vi "start_sweep.vi"(8 "error in (no error)":errorcluster, 11 "DL090130ExperimentController in":refnum<class "ExperimentControllerDL090130Interval.lvclass">) -> (0 "error out":errorcluster, 3 "DL090130ExperimentController out":refnum<class "ExperimentControllerDL090130Interval.lvclass">)   [LabVIEW 2010, in "ExperimentControllerDL090130Interval.lvclass"]
uses:
  ExperimentControllerDL090130Interval.lvclass
  ExperimentControllerDL090130Interval.lvclass/ExperimentControllerDL090130Interval.ctl
  common/classes/ErrorController/ErrorController/class_data.vi
  ImagingMode/GenericImagingMode/GenericImagingMode/GenericImagingMode.lvclass
  common/classes/ErrorController/ErrorController/ErrorController.lvclass
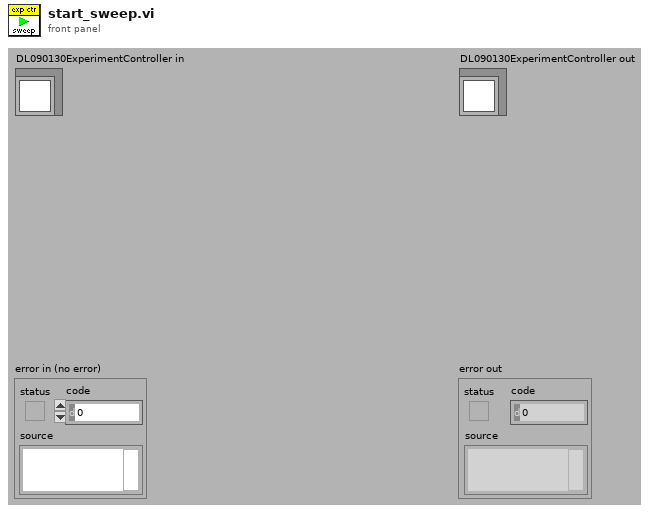
[diagram p1: front panel]
types:
  T1 = typedef "GenericToplevelComponent.lvclass/common_trigger_enum.ctl" = enum16{"NULL", "initialise", "terminate", "fetch command", "fetch data", "attach observer", "register as observer", "detach observer", "acknowledge", "start", "stop", "sweep started", "sweep finished", "experiment started", "experiment stopped"}
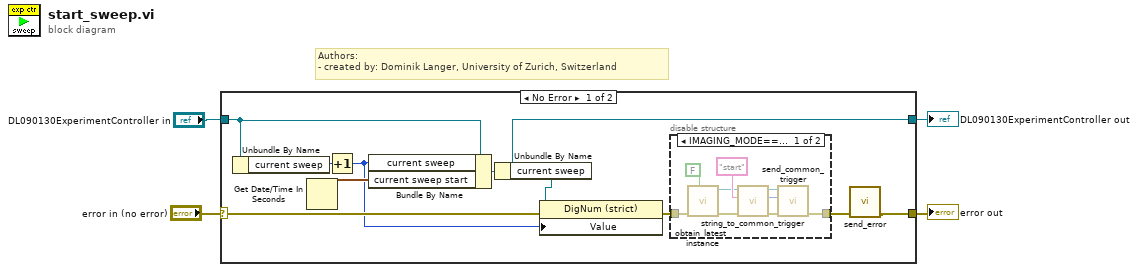
[diagram p0: block diagram]
diagram:
  # "Authors: \n- created by: Dominik Langer, University of Zurich, Switzerland"
  n1 = case shown="No Error" "error in (no error)" {
    selector: "error in (no error)" -> [w10 w26]
    tunnel: [w6 w26] -> w3
    tunnel: [w8 w25] -> w1
    tunnel: "DL090130ExperimentController in" -> [w13 w25]
    frame No Error {
      n2 = Unbundle By Name(w13) -> ("current sweep"=w14:i32)
      n3 = Get Date/Time In Seconds() -> (seconds since 1Jan1904=w12:timestamp)
      n4 = Increment(x=w14) -> (x+1=w9:i32)
      n5 = Bundle By Name(cluster=w13, "current sweep"=w9, "current sweep start"=w12) -> (w8:refnum<class "ExperimentControllerDL090130Interval.lvclass">)
      n6 = Unbundle By Name(w8) -> ("current sweep"=w11:refnum<vi>)
      n7 = property class="DigNum (strict)"(reference=w11, error in=w10, "Value"=w9) -> (error out=w7:errorcluster)  [unwired: 1 out]
      n8 = disable-structure shown="IMAGING_MODE==1" {
        disable-tunnel: w7 -> [w23 w24]
        disable-tunnel: [w22 w24] -> w5
        frame condition #0 {
          n9 = call "obtain_latest_instance.vi"("quick, but maybe outdated?"=FALSE, "error in (no error)"=w23) -> ("error out"=w19:errorcluster, "GenericScanMode out"=w17:refnum<class "GenericImagingMode.lvclass">)  [unwired: 8 in]
          n10 = call-dynamic "string_to_common_trigger.vi"("error in (no error)"=w19, "trigger string"="start", "GenericToplevelComponent in"=w17) -> ("error out"=w18:errorcluster, "trigger"=w15:T1, "GenericToplevelComponent out"=w16:refnum<class "GenericImagingMode.lvclass">)  [unwired: 6 in]
          n11 = call-dynamic "send_common_trigger.vi"("error in (no error)"=w18, "trigger"=w15, "GenericToplevelComponent in"=w16) -> ("error out"=w22:errorcluster)  [unwired: 6 in, 2 out]
        }
        frame condition #1 (active) {
        }
      }
      n12 = call "send_error.vi"("error in (no error)"=w5) -> ("error out"=w6:errorcluster)  [unwired: 10 in]
    }
    frame Error {
    }
  }
  "error out" <- w3
  "DL090130ExperimentController out" <- w1
